vi "LabVIEW -- Arduino.vi"(4 "Data to Write":u8[](array[numeric]), 5 "Frequency Write":dbl, 6 "Reset":bool, 7 "VISA resource name":refnum<visa-resource-name>) -> (0 "Read Data":u8[](array[numeric]), 1 "Read Count":i32, 2 "Write Count":u16, 3 "error IO":errorcluster)   [LabVIEW 2022 SP3]
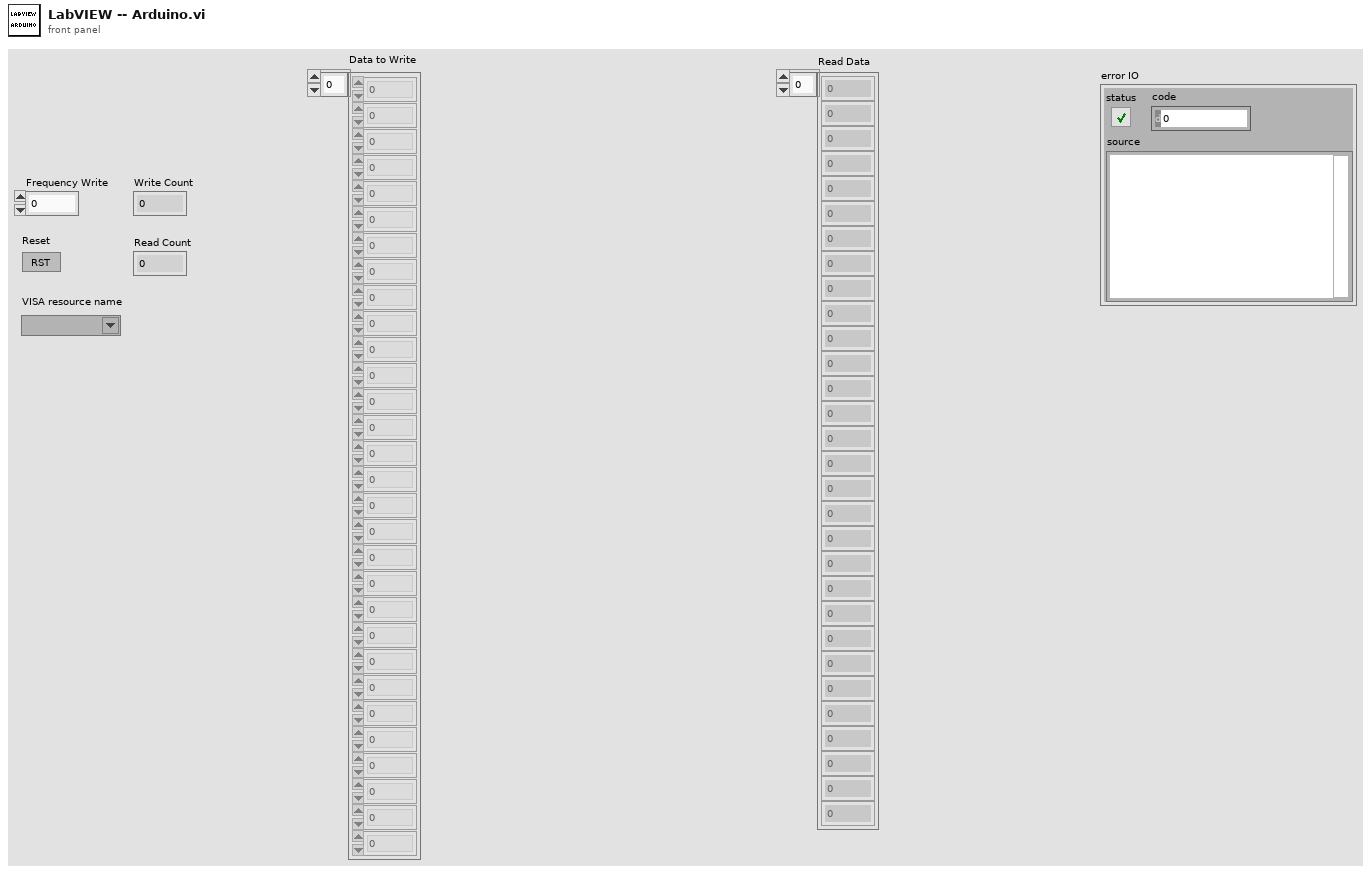
[diagram p1: front panel]
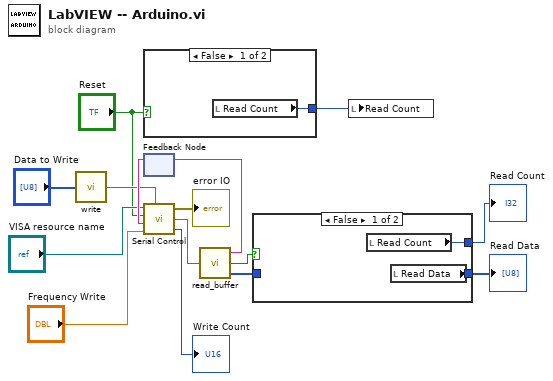
[diagram p0: block diagram]
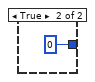
[diagram p2: hidden frame]
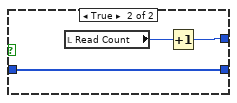
[diagram p3: hidden frame]
diagram:
  n1 = call "write.vi"("Infos"="Data to Write") -> ("to write"=w4:string)
  n2 = case shown="False" "Reset" {
    tunnel: [w16 0] -> w1
    frame False {
      n3 = local read "Read Count"() -> (w16:i32)
    }
    frame True {
    }
  }
  n4 = feedback #1() -> (w13:string)  [unwired: 1 in]
  n5 = call "Serial Control.vi"("VISA resource name"="VISA resource name", "Reset"="Reset", "Buffer_in"=w13, "Frequency Write"="Frequency Write", "write buffer"=w4) -> ("error IO"=→"error IO":errorcluster, "Buffer_out"=w11:string, "Write Count"=→"Write Count":u16)
  n6 = call "read_buffer.vi"("Buffer"=w11) -> ("Buffer Out"=w14:string, "New Packet"=w12:bool, "Data"=w6:u8[])
  n7 = feedback-in #1(w14) -> ()
  n8 = case shown="False" w12 {
    tunnel: w6 -> [_ w20]
    tunnel: [w19 w21] -> w8
    tunnel: [w18 w20] -> w7
    frame False {
      n9 = local read "Read Count"() -> (w19:i32)
      n10 = local read "Read Data"() -> (w18:u8[])
    }
    frame True {
      n11 = local read "Read Count"() -> (w22:i32)
      n12 = Increment(x=w22) -> (x+1=w21:i32)
    }
  }
  "Read Count" <- w8
  "Read Data" <- w7
  n13 = local write "Read Count"(w1) -> ()
